vi "Type.vi"(11 "Module in":refnum<class "Module.lvclass">) -> (2 "Module Type":string, 3 "Module out":refnum<class "Module.lvclass">)   [LabVIEW 2020, in "Volatus.lvlib" / "Module.lvclass"]
uses:
  Module.lvclass
  Module.lvclass/Module.ctl
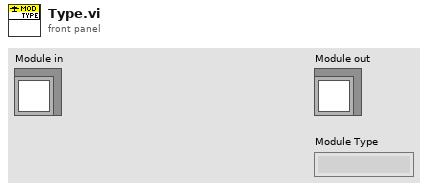
[diagram p1: front panel]
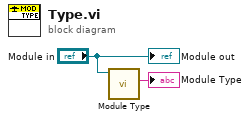
[diagram p0: block diagram]
diagram:
  n1 = call-dynamic "Module Type.vi"("Module in"="Module in") -> ("Module Type"=→"Module Type":string)  [unwired: 10 in]
  "Module out" <- "Module in"
